vi "ANAL_AddData.vi"(9 "Run Data Cluster In":T3 {"Temperature B" scale=0.0..100.0; "Temperature A" scale=0.0..100.0}, 10 "Run Info In":T2, 11 "Main Data Array":T1 {"Run Data Cluster"."Temperature B" scale=0.0..100.0; "Run Data Cluster"."Temperature A" scale=0.0..100.0}) -> (0 "ID":u32, 3 "output array":T1 {"Run Data Cluster"."Temperature B" scale=0.0..100.0; "Run Data Cluster"."Temperature A" scale=0.0..100.0})   [LabVIEW 2021]
uses:
  ANAL_Data.ctl
  XML_Cluster.ctl
  DAT_Cluster.ctl
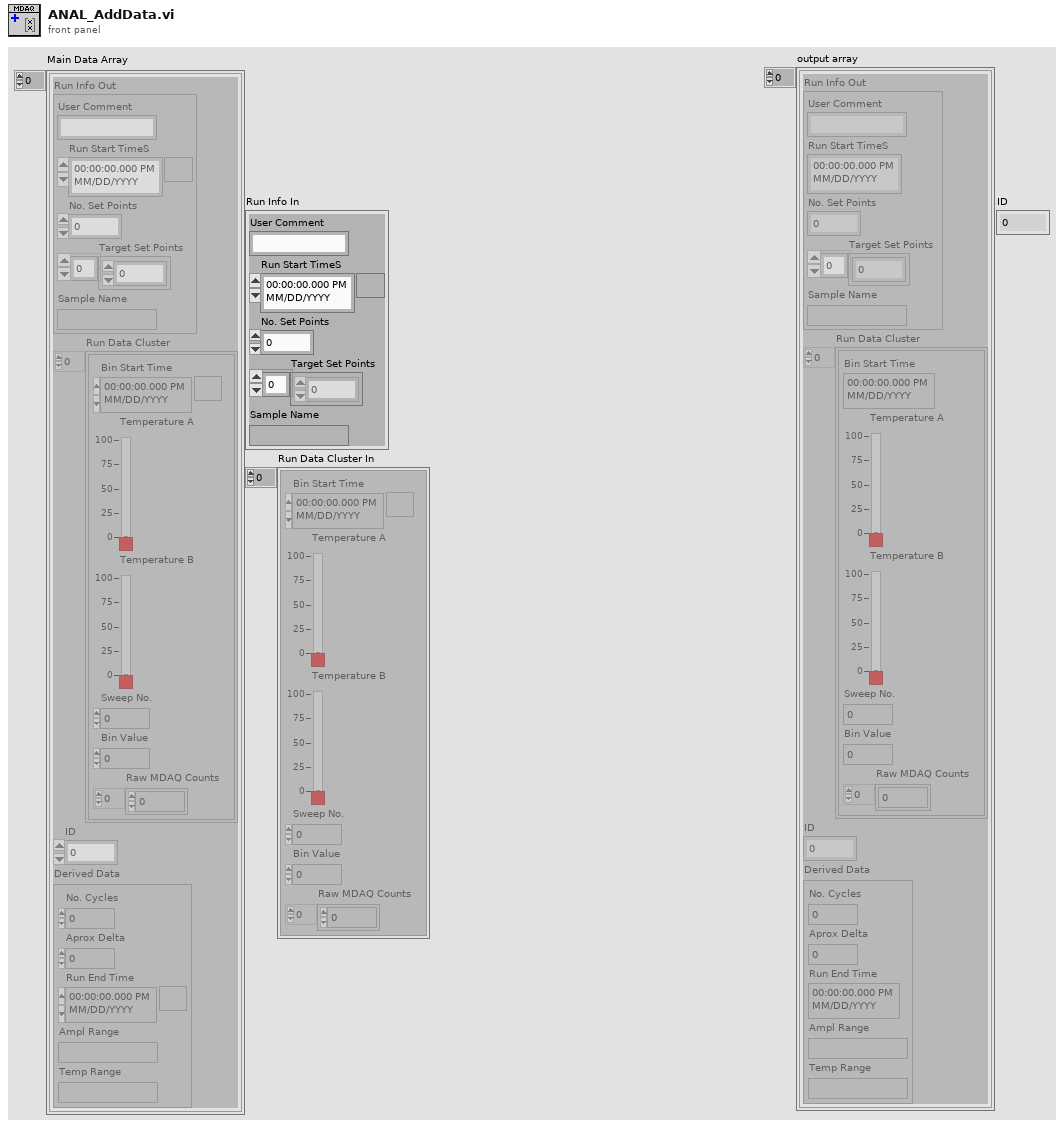
[diagram p1: front panel]
types:
  T1 = typedef "ANAL_Data.ctl" = cluster{"Run Info Out":T2, "Run Data Cluster":T3, "ID":u32, "Derived Data":cluster{"No. Cycles":u32, "Aprox Delta":dbl, "Run End Time":timestamp, "Ampl Range":string, "Temp Range":string}}[]
  T2 = typedef "XML_Cluster.ctl" = cluster{"User Comment":string, "Run Start TimeS":timestamp, "No. Set Points":u32, "Target Set Points":i32[], "Sample Name":string}
  T3 = typedef "DAT_Cluster.ctl" = cluster{"Bin Start Time":timestamp, "Temperature A":dbl, "Temperature B":dbl, "Sweep No.":i32, "Bin Value":i32, "Raw MDAQ Counts":i32[]}[]
  T4 = cluster{"Run Info Out":T2, "Run Data Cluster":T3, "ID":u32, "Derived Data":cluster{"No. Cycles":u32, "Aprox Delta":dbl, "Run End Time":timestamp, "Ampl Range":string, "Temp Range":string}}
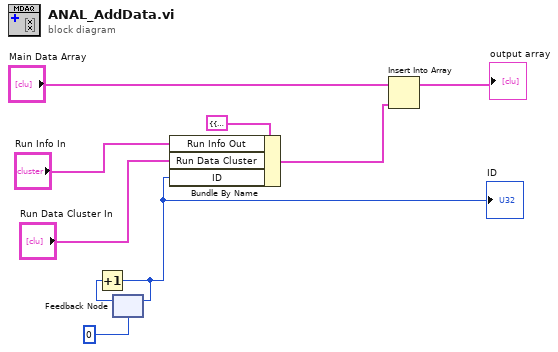
[diagram p0: block diagram]
diagram:
  n1 = feedback #1(u32 0) -> (w4:u32)
  n2 = Increment(x=w4) -> (x+1=w3:u32)
  "ID" <- w3
  n3 = feedback-in #1(w3) -> ()
  n4 = Bundle By Name(cluster=T4 {"Run Info Out"={"User Comment"="", "Run Start TimeS"=timestamp(0 s since 1904-01-01), "No. Set Points"=0, "Target Set Points"=[], "Sample Name"=""}, "Run Data Cluster"=[], "ID"=0, "Derived Data"={"No. Cycles"=0, "Aprox Delta"=0.0, "Run End Time"=timestamp(0 s since 1904-01-01), "Ampl Range"="", "Temp Range"=""}} ("new element/subarray"), "Run Info Out"="Run Info In", "Run Data Cluster"="Run Data Cluster In", "ID"=w3) -> (w1:T4)
  n5 = Insert Into Array(array="Main Data Array", new element=w1) -> (→"output array":T1)  [unwired: 1 in]
